vi "ClearFP.vi"(8 "error in (no error)":errorcluster, 9 "ConPaneMode?":bool=TRUE, 10 "ProjectItemRef":refnum<vi>, 11 "CS++Actor in":refnum<class "CS++Actor.lvclass">) -> (0 "error out":errorcluster, 3 "CS++Actor out":refnum<class "CS++Actor.lvclass">)   [LabVIEW 2016, in "CS++Actor.lvlib" / "CS++Actor.lvclass"]
doc: "This VI resets FP elements. All controls will be on the left side, all indicators on the right side."
uses:
  CS++Actor.lvclass
  <vilib>/Utility/traverseref.llb/TRef TravTarget.ctl
  <vilib>/Utility/miscctls.llb/LVRectTypeDef.ctl
  <vilib>/Utility/VariantDataType/Type.ctl
  <vilib>/Utility/VariantDataType/VariantType.lvlib
  <vilib>/Utility/Data Type/NI_Data Type.lvlib
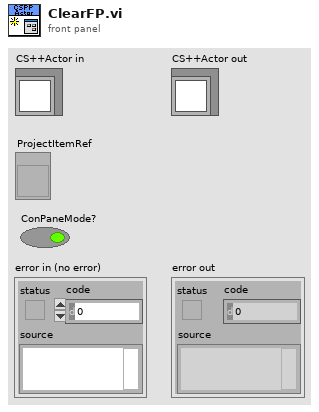
[diagram p1: front panel]
types:
  T1 = enum16{"Invalid Wire Rule", "Required", "Recommended", "Optional", "Dynamic Dispatch"}
  T2 = enum32{"Top Edges", "Vertical Centers", "Bottom Edges", "Left Edges", "Horizontal Centers", "Right Edges"}
  T3 = enum32{"Top Edges", "Vertical Centers", "Bottom Edges", "Vertical Gap", "Vertical Compress", "Left Edges", "Horizontal Centers", "Right Edges", "Horizontal Gap", "Horizontal Compress"}
  T4 = typedef "TRef TravTarget.ctl" = enum16{"FP", "BD", "Other"}
  T5 = typedef "LVRectTypeDef.ctl" = cluster{"Left":i16, "Top":i16, "Right":i16, "Bottom":i16}
  T6 = typedef "VariantType.lvlib/Type.ctl" = enum8{"Invalid Type", "Void", "I8", "I16", "I32", "I64", "U8", "U16", "U32", "U64", "Single Float", "Double Float", "Extended Float", "Single Complex", "Double Complex", "Extended Complex", "Enum U8", "Enum U16", "Enum U32", "Enum U64", "Single Float With Unit", "Double Float With Unit", "Extended Float With Unit", "Single Complex with Unit", "Double Complex with Unit", "Extended Complex with Unit", "Boolean", "String", "Path", "Picture", "Tag", "Array", "Cluster", "Variant", "LV Variant", "Waveform", "Timestamp", "Digital Waveform", "Digital Data", "ExpressData", "Refnum", "External Data", "VI", "Poly VI", "LabVIEW Class Instance", "Fixed Point"}
  T7 = enum16{"Invalid Wire Rule", "Required", "Recommended", "Optional", "Dynamic Dispatch"}[]
  T8 = typedef "NI_Data Type.lvlib/Data Type.ctl" = enum8{"Invalid Type", "Void", "I8", "I16", "I32", "I64", "U8", "U16", "U32", "U64", "Single Float", "Double Float", "Extended Float", "Single Complex", "Double Complex", "Extended Complex", "Enum U8", "Enum U16", "Enum U32", "Enum U64", "Single Float With Unit", "Double Float With Unit", "Extended Float With Unit", "Single Complex with Unit", "Double Complex with Unit", "Extended Complex with Unit", "Boolean", "String", "Path", "Picture", "Tag", "Array", "Cluster", "Variant", "LV Variant", "Waveform", "Timestamp", "Digital Waveform", "Digital Data", "ExpressData", "Refnum", "External Data", "VI", "Poly VI", "LabVIEW Class Instance", "Fixed Point"}
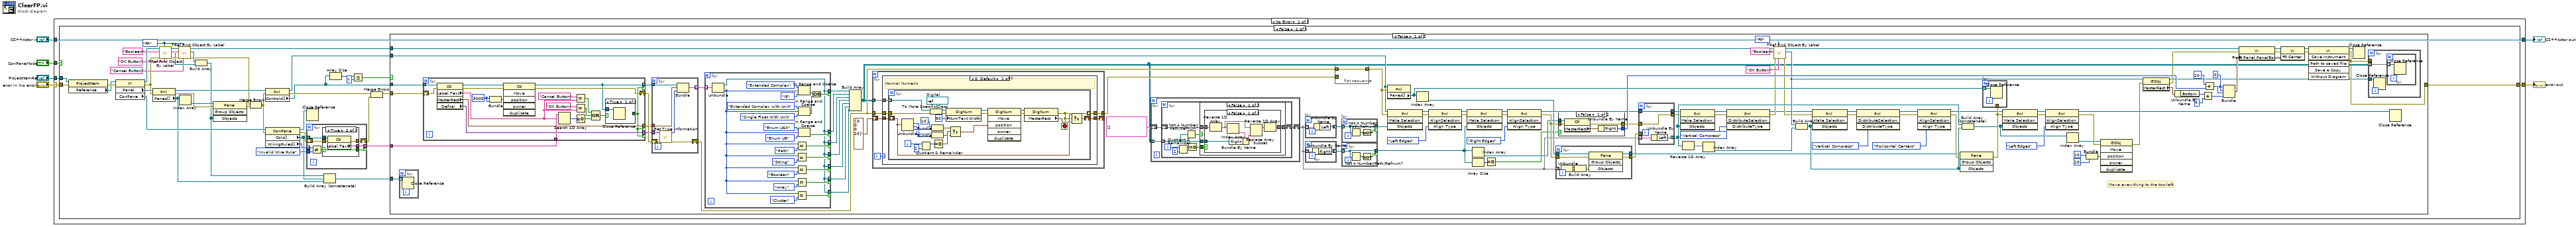
[diagram p0: block diagram]
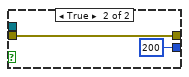
[diagram p2: hidden frame]
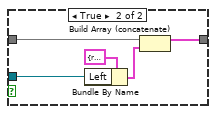
[diagram p3: hidden frame]
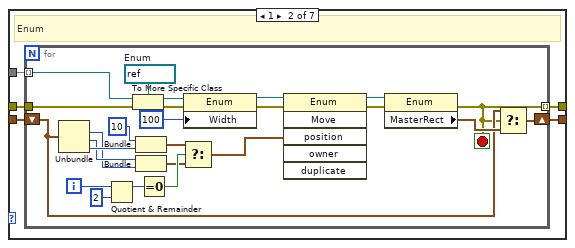
[diagram p5: hidden frame]
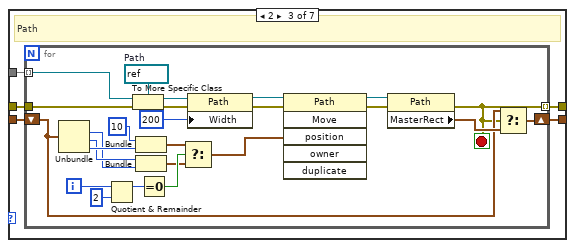
[diagram p6: hidden frame]
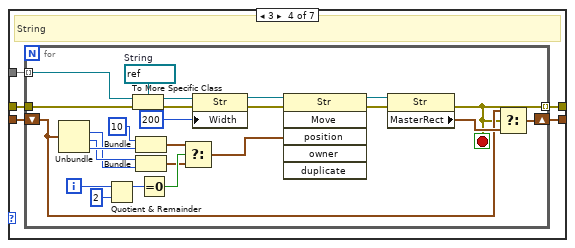
[diagram p7: hidden frame]
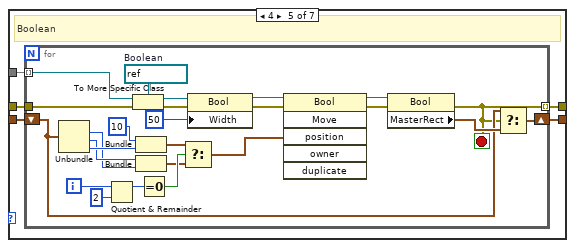
[diagram p8: hidden frame]
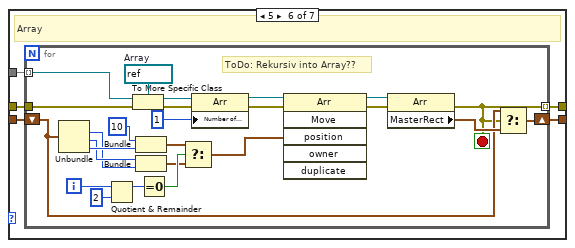
[diagram p9: hidden frame]
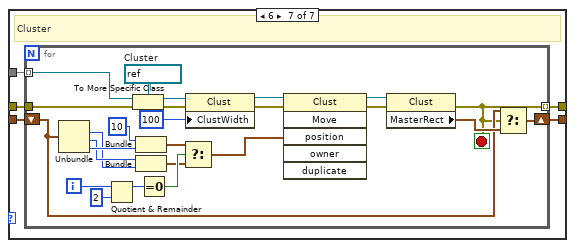
[diagram p10: hidden frame]
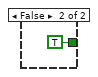
[diagram p11: hidden frame]
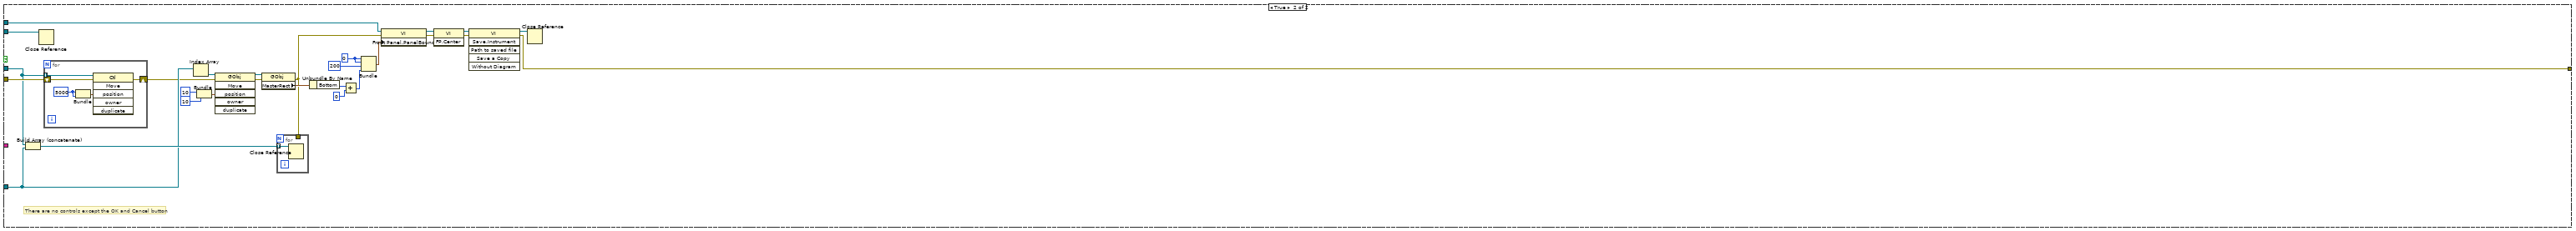
[diagram p12: hidden frame]
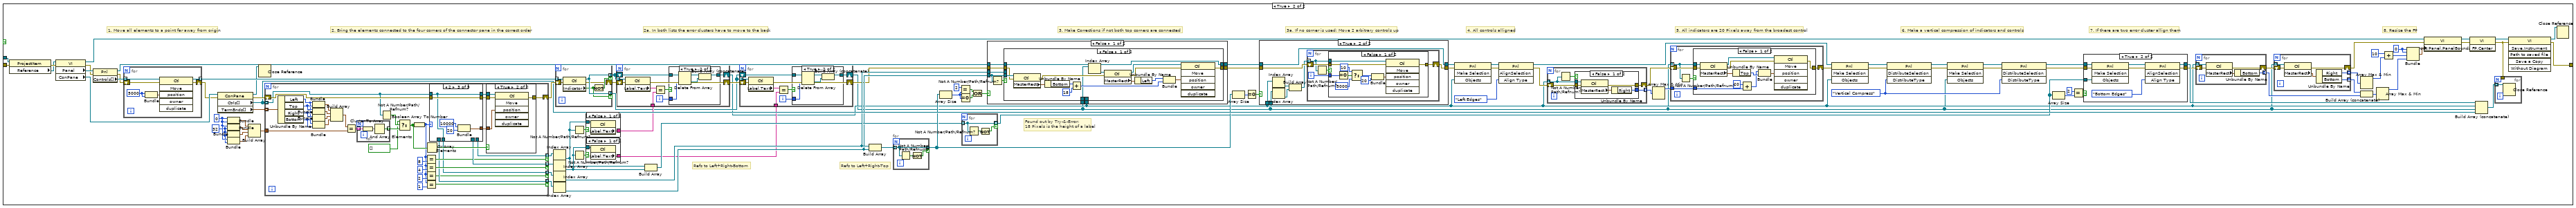
[diagram p14: hidden frame]
diagram:
  n1 = case shown="No Error" "error in (no error)" {
    selector: "error in (no error)" -> [w9 w872]
    tunnel: [w10 w872] -> w5
    tunnel: [w11 w871] -> w3
    tunnel: "CS++Actor in" -> [w11 w871]
    tunnel: "ProjectItemRef" -> [w8 _]
    tunnel: "ConPaneMode?" -> [w7 _]
    frame No Error {
      n2 = case shown="False" w7 {
        tunnel: [w42 w577] -> w10
        tunnel: w9 -> [w40 w576]
        tunnel: w8 -> [w41 w573]
        frame False {
          w31 = "Boolean" ("Class Name")
          w32 = TRef_TravTarget."FP" ("Traverse Target")
          n3 = property class="ProjectItem"(reference=w41, error in=w40) -> (error out=w39:errorcluster, "Reference"=w38:refnum<vi>)  [unwired: 1 out]
          n4 = property class="VI"(reference=w38, error in=w39) -> (reference out=w37:refnum<vi>, error out=w23:errorcluster, "Panel"=w29:refnum<vi>, "ConPane"=w43:refnum<vi>)
          n5 = property class="Pnl"(reference=w29, error in=w23) -> (reference out=w28:refnum<vi>, error out=w26:errorcluster, "Panes[]"=w19:refnum<vi>[])
          n6 = call <vilib>:"TRef Find Object By Label.vi"("Label"="OK Button", "Traverse Target"=w32, "error in (no error)"=w23, "Class Name"=w31, "VI Ref"=w37) -> ("error out"=w33:errorcluster, "Found Obj Ref"=w24:refnum<vi>, "dup VI Ref"=w35:refnum<vi>)  [unwired: 3 in, 1 out]
          n7 = call <vilib>:"TRef Find Object By Label.vi"("Label"="Cancel Button", "Traverse Target"=w32, "error in (no error)"=w33, "Class Name"=w31, "VI Ref"=w35) -> ("error out"=w21:errorcluster, "Found Obj Ref"=w25:refnum<vi>, "dup VI Ref"=w34:refnum<vi>)  [unwired: 3 in, 1 out]
          n8 = Index Array(array=w19) -> (element=w27:refnum<vi>)  [unwired: 1 in]
          n9 = Build Array(w25, w24) -> (w13:refnum<vi>[])
          n10 = invoke class="Pane" method="Group Objects"(reference=w27, error in=w26, "Objects"=w13) -> (error out=w22:errorcluster)  [unwired: 1 in, 3 out]
          n11 = Merge Errors(w21, w22) -> (w20:errorcluster)
          n12 = property class="Pnl"(reference=w28, error in=w20) -> (reference out=w51:refnum<vi>, error out=w45:errorcluster, "Controls[]"=w18:refnum<vi>[])
          n13 = property class="ConPane"(reference=w43, error in=w20) -> (reference out=w48:refnum<vi>, error out=w44:errorcluster, "Ctrls[]"=w12:refnum<vi>[], "WiringRules[]"=w49:T7)
          n14 = Close Reference(reference=w48) -> ()  [unwired: 1 in, 1 out]
          n15 = for {
            tunnel: w12 -> [w525] mode=indexing
            shift-right: [w523] -> w47
            shift-left: w44 -> [w524]
            tunnel: [w522] -> w52 mode=indexing if=w518
            tunnel: w49 -> [w520] mode=indexing
            tunnel: T1."Invalid Wire Rule" ("Wire Rule") -> [w519]
            n16 = Not Equal?(x=w520, y=w519) -> (x != y?=w521:bool)
            n17 = case shown="True" w521 {
              selector: w521 -> [w526 w528]
              tunnel: w525 -> [_ w532]
              tunnel: w524 -> [w527 w531]
              tunnel: [w527 w530] -> w523
              tunnel: [_ w529] -> w522
              tunnel: [w526 w528] -> w518
              frame False {
              }
              frame True {
                n18 = property class="Ctl"(reference=w532, error in=w531) -> (error out=w530:errorcluster, "Label.Text"=w529:string)  [unwired: 1 out]
              }
            }
          }
          n19 = Build Array (concatenate)(w13, w12, w19) -> (w14:refnum<vi>[])
          n20 = Array Size(array=w18) -> (size(s)=w17:i32)
          n21 = Less Or Equal?(x=w17, y=7) -> (x <= y?=w15:bool)
          n22 = Merge Errors(w45, w47) -> (w46:errorcluster)
          n23 = case shown="False" w15 {
            tunnel: w52 -> [w148 _]
            tunnel: w51 -> [w100 w492]
            tunnel: w46 -> [w71 w487]
            tunnel: [w70 w490] -> w42
            tunnel: w34 -> [w55 w496]
            tunnel: w18 -> [w54 w485]
            tunnel: w14 -> [w53 w488]
            frame False {
              w140 = i16 0 ("y")
              # "Move everything to the top-left"
              n24 = for {
                tunnel: w53 -> [w154] mode=indexing
                n25 = Close Reference(reference=w154) -> ()  [unwired: 1 in, 1 out]
              }
              n26 = for {
                tunnel: w54 -> [w482] mode=indexing
                shift-right: [w474] -> w75
                shift-left: w71 -> [w481]
                tunnel: w148 -> [w480]
                tunnel: [w475] -> w74 mode=indexing if=w471
                tunnel: [w473] -> w73 mode=indexing if=w471
                tunnel: [w472] -> w72 mode=indexing if=w471
                w479 = i16 5000 ("x")
                n27 = property class="Ctl"(reference=w482, error in=w481) -> (reference out=w476:refnum<vi>, error out=w477:errorcluster, "Label.Text"=w469:string, "MasterRect"=w473:T5, "DefVal"=w472:variant)
                n28 = Bundle("x"=w479, "x"=w479) -> (w478:cluster{"x":i16, "x":i16})  [unwired: 1 in]
                n29 = invoke class="Ctl" method="Move"(reference=w476, error in=w477, "position"=w478) -> (reference out=w475:refnum<vi>, error out=w474:errorcluster)  [unwired: 3 in, 4 out]
                n30 = Search 1D Array(1D array=w480, element=w469) -> (index of element=w470:i32)  [unwired: 1 in]
                n31 = Equal?(x="Cancel Button", y=w469) -> (x = y?=w468:bool)
                n32 = Equal?(x="OK Button", y=w469) -> (x = y?=w467:bool)
                n33 = Greater Or Equal To 0?(x=w470) -> (x >= 0?=w466:bool)
                n34 = Compound Arithmetic op=OR(w468, w467, w466) -> (w465:bool)
                n35 = case shown="True" w465 {
                  tunnel: w475 -> [w483 _]
                  tunnel: [_ TRUE] -> w471
                  frame True {
                    n36 = Close Reference(reference=w483) -> ()  [unwired: 1 in, 1 out]
                  }
                  frame False {
                  }
                }
              }
              n37 = for {
                tunnel: w72 -> [w462] mode=indexing
                tunnel: w73 -> [w460] mode=indexing
                tunnel: w74 -> [w461] mode=indexing
                tunnel: [w459] -> w76 mode=indexing
                shift-right: [w457] -> w98
                shift-left: w75 -> [w458]
                n38 = call <vilib>:"Get Type Information.vi"("error in (no error)"=w458, "Variant"=w462) -> ("error out"=w457:errorcluster, "Type"=w456:T8)  [unwired: 5 in, 3 out]
                n39 = Bundle(w461, "MasterRect"=w460, "Type"=w456) -> (w459:cluster{refnum<vi>, "MasterRect":T5, "Type":T8})  [unwired: 1 in]
              }
              n40 = for {
                tunnel: w76 -> [w435] mode=indexing
                tunnel: [w433] -> w77 mode=indexing if=w449
                tunnel: [w433] -> w78 mode=indexing if=w446
                tunnel: [w433] -> w79 mode=indexing if=w436
                tunnel: [w433] -> w82 mode=indexing if=w444
                tunnel: [w433] -> w83 mode=indexing if=w441
                tunnel: [w433] -> w84 mode=indexing if=w440
                tunnel: [w433] -> w81 mode=indexing if=w434
                n41 = Unbundle(w435) -> (w433:refnum<vi>, "Type"=w437:T8)  [unwired: 1 out]
                n42 = Equal?(x=w437, y=Type."Path" ("Type Enum")) -> (x = y?=w436:bool)
                n43 = Equal?(x=w437, y=Type."String" ("Type Enum")) -> (x = y?=w434:bool)
                n44 = Equal?(x=w437, y=Type."Boolean" ("Type Enum")) -> (x = y?=w444:bool)
                n45 = Equal?(x=w437, y=Type."Array" ("Type Enum")) -> (x = y?=w441:bool)
                n46 = Equal?(x=w437, y=Type."Cluster" ("Type Enum")) -> (x = y?=w440:bool)
                n47 = In Range and Coerce(upper limit=Type."Extended Complex" ("Type Enum"), x=w437, lower limit=Type."I8" ("Type Enum")) -> (In Range?=w451:bool)  [unwired: 1 out]
                n48 = In Range and Coerce(upper limit=Type."Extended Complex with Unit" ("Type Enum"), x=w437, lower limit=Type."Single Float With Unit" ("Type Enum")) -> (In Range?=w450:bool)  [unwired: 1 out]
                n49 = In Range and Coerce(upper limit=Type."Enum U64" ("Type Enum"), x=w437, lower limit=Type."Enum U8" ("Type Enum")) -> (In Range?=w446:bool)  [unwired: 1 out]
                n50 = Or(x=w451, y=w450) -> (x .or. y?=w449:bool)
              }
              n51 = Build Array(w77, w78, w79, w81, w82, w83, w84) -> (w85:refnum<vi>[][])
              n52 = for {
                tunnel: w85 -> [w221] mode=indexing
                shift-right: [w218] -> _
                shift-left: T5 {"Left"=0, "Top"=0, "Right"=0, "Bottom"=20} ("MasterRect") -> [w219]
                tunnel: w98 -> [w222]
                tunnel: [w217] -> w99 mode=concatenating
                i -> [w220]
                n53 = case shown="0, Default" w220 {
                  tunnel: w221 -> [w227 w257 w287 w317 w347 w377 w407]
                  tunnel: [w226 w256 w286 w316 w346 w376 w406] -> w217
                  tunnel: [w225 w255 w285 w315 w345 w375 w405] -> w218
                  tunnel: w222 -> [w224 w254 w284 w314 w344 w374 w404]
                  tunnel: w219 -> [w223 w253 w283 w313 w343 w373 w403]
                  frame 0, Default {
                    # "Normal Numeric"
                    n54 = for {
                      tunnel: w227 -> [w232] mode=indexing
                      shift-right: [w231] -> w225
                      shift-left: w223 -> [w229]
                      tunnel: w224 -> [w251]
                      tunnel: [w228] -> w226 mode=indexing
                      i -> [w252]
                      stop <- w228 stop-if-true
                      w233 = refnum<vi> refnum  # Digital
                      n55 = Unbundle(w229) -> ("Top"=w234:i16, "Right"=w235:i16, "Bottom"=w236:i16)  [unwired: 1 out]
                      n56 = Quotient & Remainder(x=w252, y=2) -> (x-y*floor(x/y)=w242:i32)  [unwired: 1 out]
                      n57 = To More Specific Class(target class=w233, reference=w232, error in=w251) -> (specific class reference=w249:refnum<vi>, error out=w248:errorcluster)
                      n58 = Bundle("Top"=i16 10, "Bottom"=w236) -> (w239:cluster{"Top":i16, "Bottom":i16})  [unwired: 1 in]
                      n59 = Bundle("Right"=w235, "Top"=w234) -> (w238:cluster{"Right":i16, "Top":i16})  [unwired: 1 in]
                      n60 = Equal To 0?(x=w242) -> (x = 0?=w241:bool)
                      n61 = property class="DigNum"(reference=w249, error in=w248, "NumText.Width"=u32 50 ("Numeric Text.Size:Width")) -> (reference out=w247:refnum<vi>, error out=w246:errorcluster)
                      n62 = Select(t=w239, s=w241, f=w238) -> (s? t:f=w240:cluster{"Right":i16, "Top":i16})
                      n63 = invoke class="DigNum" method="Move"(reference=w247, error in=w246, "position"=w240) -> (reference out=w244:refnum<vi>, error out=w243:errorcluster)  [unwired: 3 in, 4 out]
                      n64 = property class="DigNum"(reference=w244, error in=w243) -> (error out=w228:errorcluster, "MasterRect"=w230:T5)  [unwired: 1 out]
                      n65 = Select(t=w229, s=w228, f=w230) -> (s? t:f=w231:T5)
                    }
                  }
                  frame 1 {
                    # "Enum"
                    n66 = for {
                      tunnel: w257 -> [w262] mode=indexing
                      shift-right: [w261] -> w255
                      shift-left: w253 -> [w259]
                      tunnel: w254 -> [w281]
                      tunnel: [w258] -> w256 mode=indexing
                      i -> [w282]
                      stop <- w258 stop-if-true
                      w263 = refnum<vi> refnum  # Enum
                      n67 = Unbundle(w259) -> ("Top"=w264:i16, "Right"=w265:i16, "Bottom"=w266:i16)  [unwired: 1 out]
                      n68 = Quotient & Remainder(x=w282, y=2) -> (x-y*floor(x/y)=w272:i32)  [unwired: 1 out]
                      n69 = To More Specific Class(target class=w263, reference=w262, error in=w281) -> (specific class reference=w279:refnum<vi>, error out=w278:errorcluster)
                      n70 = Bundle("Top"=i16 10, "Bottom"=w266) -> (w269:cluster{"Top":i16, "Bottom":i16})  [unwired: 1 in]
                      n71 = Bundle("Right"=w265, "Top"=w264) -> (w268:cluster{"Right":i16, "Top":i16})  [unwired: 1 in]
                      n72 = Equal To 0?(x=w272) -> (x = 0?=w271:bool)
                      n73 = Select(t=w269, s=w271, f=w268) -> (s? t:f=w270:cluster{"Right":i16, "Top":i16})
                      n74 = property class="Enum"(reference=w279, error in=w278, "Width"=u32 100 ("Numeric Text.Size:Width")) -> (reference out=w277:refnum<vi>, error out=w276:errorcluster)
                      n75 = invoke class="Enum" method="Move"(reference=w277, error in=w276, "position"=w270) -> (reference out=w274:refnum<vi>, error out=w273:errorcluster)  [unwired: 3 in, 4 out]
                      n76 = property class="Enum"(reference=w274, error in=w273) -> (error out=w258:errorcluster, "MasterRect"=w260:T5)  [unwired: 1 out]
                      n77 = Select(t=w259, s=w258, f=w260) -> (s? t:f=w261:T5)
                    }
                  }
                  frame 2 {
                    # "Path"
                    n78 = for {
                      tunnel: w287 -> [w292] mode=indexing
                      shift-right: [w291] -> w285
                      shift-left: w283 -> [w289]
                      tunnel: w284 -> [w311]
                      tunnel: [w288] -> w286 mode=indexing
                      i -> [w312]
                      stop <- w288 stop-if-true
                      w293 = refnum<vi> refnum  # Path
                      n79 = Unbundle(w289) -> ("Top"=w294:i16, "Right"=w295:i16, "Bottom"=w296:i16)  [unwired: 1 out]
                      n80 = Quotient & Remainder(x=w312, y=2) -> (x-y*floor(x/y)=w302:i32)  [unwired: 1 out]
                      n81 = To More Specific Class(target class=w293, reference=w292, error in=w311) -> (specific class reference=w309:refnum<vi>, error out=w308:errorcluster)
                      n82 = Bundle("Top"=i16 10, "Bottom"=w296) -> (w299:cluster{"Top":i16, "Bottom":i16})  [unwired: 1 in]
                      n83 = Bundle("Right"=w295, "Top"=w294) -> (w298:cluster{"Right":i16, "Top":i16})  [unwired: 1 in]
                      n84 = Equal To 0?(x=w302) -> (x = 0?=w301:bool)
                      n85 = Select(t=w299, s=w301, f=w298) -> (s? t:f=w300:cluster{"Right":i16, "Top":i16})
                      n86 = property class="Path"(reference=w309, error in=w308, "Width"=u32 200 ("Numeric Text.Size:Width")) -> (reference out=w307:refnum<vi>, error out=w306:errorcluster)
                      n87 = invoke class="Path" method="Move"(reference=w307, error in=w306, "position"=w300) -> (reference out=w304:refnum<vi>, error out=w303:errorcluster)  [unwired: 3 in, 4 out]
                      n88 = property class="Path"(reference=w304, error in=w303) -> (error out=w288:errorcluster, "MasterRect"=w290:T5)  [unwired: 1 out]
                      n89 = Select(t=w289, s=w288, f=w290) -> (s? t:f=w291:T5)
                    }
                  }
                  frame 3 {
                    # "String"
                    n90 = for {
                      tunnel: w317 -> [w322] mode=indexing
                      shift-right: [w321] -> w315
                      shift-left: w313 -> [w319]
                      tunnel: w314 -> [w341]
                      tunnel: [w318] -> w316 mode=indexing
                      i -> [w342]
                      stop <- w318 stop-if-true
                      w323 = refnum<vi> refnum  # String
                      n91 = Unbundle(w319) -> ("Top"=w324:i16, "Right"=w325:i16, "Bottom"=w326:i16)  [unwired: 1 out]
                      n92 = Quotient & Remainder(x=w342, y=2) -> (x-y*floor(x/y)=w332:i32)  [unwired: 1 out]
                      n93 = To More Specific Class(target class=w323, reference=w322, error in=w341) -> (specific class reference=w339:refnum<vi>, error out=w338:errorcluster)
                      n94 = Bundle("Top"=i16 10, "Bottom"=w326) -> (w329:cluster{"Top":i16, "Bottom":i16})  [unwired: 1 in]
                      n95 = Bundle("Right"=w325, "Top"=w324) -> (w328:cluster{"Right":i16, "Top":i16})  [unwired: 1 in]
                      n96 = Equal To 0?(x=w332) -> (x = 0?=w331:bool)
                      n97 = Select(t=w329, s=w331, f=w328) -> (s? t:f=w330:cluster{"Right":i16, "Top":i16})
                      n98 = property class="Str"(reference=w339, error in=w338, "Width"=u32 200 ("Numeric Text.Size:Width")) -> (reference out=w337:refnum<vi>, error out=w336:errorcluster)
                      n99 = invoke class="Str" method="Move"(reference=w337, error in=w336, "position"=w330) -> (reference out=w334:refnum<vi>, error out=w333:errorcluster)  [unwired: 3 in, 4 out]
                      n100 = property class="Str"(reference=w334, error in=w333) -> (error out=w318:errorcluster, "MasterRect"=w320:T5)  [unwired: 1 out]
                      n101 = Select(t=w319, s=w318, f=w320) -> (s? t:f=w321:T5)
                    }
                  }
                  frame 4 {
                    # "Boolean"
                    n102 = for {
                      tunnel: w347 -> [w352] mode=indexing
                      shift-right: [w351] -> w345
                      shift-left: w343 -> [w349]
                      tunnel: w344 -> [w371]
                      tunnel: [w348] -> w346 mode=indexing
                      i -> [w372]
                      stop <- w348 stop-if-true
                      w353 = refnum<vi> refnum  # Boolean
                      n103 = Unbundle(w349) -> ("Top"=w354:i16, "Right"=w355:i16, "Bottom"=w356:i16)  [unwired: 1 out]
                      n104 = Quotient & Remainder(x=w372, y=2) -> (x-y*floor(x/y)=w362:i32)  [unwired: 1 out]
                      n105 = To More Specific Class(target class=w353, reference=w352, error in=w371) -> (specific class reference=w369:refnum<vi>, error out=w368:errorcluster)
                      n106 = Bundle("Top"=i16 10, "Bottom"=w356) -> (w359:cluster{"Top":i16, "Bottom":i16})  [unwired: 1 in]
                      n107 = Bundle("Right"=w355, "Top"=w354) -> (w358:cluster{"Right":i16, "Top":i16})  [unwired: 1 in]
                      n108 = Equal To 0?(x=w362) -> (x = 0?=w361:bool)
                      n109 = Select(t=w359, s=w361, f=w358) -> (s? t:f=w360:cluster{"Right":i16, "Top":i16})
                      n110 = property class="Bool"(reference=w369, error in=w368, "Width"=u32 50 ("Numeric Text.Size:Width")) -> (reference out=w367:refnum<vi>, error out=w366:errorcluster)
                      n111 = invoke class="Bool" method="Move"(reference=w367, error in=w366, "position"=w360) -> (reference out=w364:refnum<vi>, error out=w363:errorcluster)  [unwired: 3 in, 4 out]
                      n112 = property class="Bool"(reference=w364, error in=w363) -> (error out=w348:errorcluster, "MasterRect"=w350:T5)  [unwired: 1 out]
                      n113 = Select(t=w349, s=w348, f=w350) -> (s? t:f=w351:T5)
                    }
                  }
                  frame 5 {
                    # "Array"
                    n114 = for {
                      tunnel: w377 -> [w382] mode=indexing
                      shift-right: [w381] -> w375
                      shift-left: w373 -> [w379]
                      tunnel: w374 -> [w401]
                      tunnel: [w378] -> w376 mode=indexing
                      i -> [w402]
                      stop <- w378 stop-if-true
                      w383 = refnum<vi> refnum  # Array
                      # "ToDo: Rekursiv into Array??"
                      n115 = Unbundle(w379) -> ("Top"=w384:i16, "Right"=w385:i16, "Bottom"=w386:i16)  [unwired: 1 out]
                      n116 = Quotient & Remainder(x=w402, y=2) -> (x-y*floor(x/y)=w392:i32)  [unwired: 1 out]
                      n117 = To More Specific Class(target class=w383, reference=w382, error in=w401) -> (specific class reference=w399:refnum<vi>, error out=w398:errorcluster)
                      n118 = Bundle("Top"=i16 10, "Bottom"=w386) -> (w389:cluster{"Top":i16, "Bottom":i16})  [unwired: 1 in]
                      n119 = Bundle("Right"=w385, "Top"=w384) -> (w388:cluster{"Right":i16, "Top":i16})  [unwired: 1 in]
                      n120 = Equal To 0?(x=w392) -> (x = 0?=w391:bool)
                      n121 = Select(t=w389, s=w391, f=w388) -> (s? t:f=w390:cluster{"Right":i16, "Top":i16})
                      n122 = property class="Arr"(reference=w399, error in=w398, "Number of Columns"=u32 1 ("Numeric Text.Size:Width")) -> (reference out=w397:refnum<vi>, error out=w396:errorcluster)
                      n123 = invoke class="Arr" method="Move"(reference=w397, error in=w396, "position"=w390) -> (reference out=w394:refnum<vi>, error out=w393:errorcluster)  [unwired: 3 in, 4 out]
                      n124 = property class="Arr"(reference=w394, error in=w393) -> (error out=w378:errorcluster, "MasterRect"=w380:T5)  [unwired: 1 out]
                      n125 = Select(t=w379, s=w378, f=w380) -> (s? t:f=w381:T5)
                    }
                  }
                  frame 6 {
                    # "Cluster"
                    n126 = for {
                      tunnel: w407 -> [w412] mode=indexing
                      shift-right: [w411] -> w405
                      shift-left: w403 -> [w409]
                      tunnel: w404 -> [w431]
                      tunnel: [w408] -> w406 mode=indexing
                      i -> [w432]
                      stop <- w408 stop-if-true
                      w413 = refnum<vi> refnum  # Cluster
                      n127 = Unbundle(w409) -> ("Top"=w414:i16, "Right"=w415:i16, "Bottom"=w416:i16)  [unwired: 1 out]
                      n128 = Quotient & Remainder(x=w432, y=2) -> (x-y*floor(x/y)=w422:i32)  [unwired: 1 out]
                      n129 = To More Specific Class(target class=w413, reference=w412, error in=w431) -> (specific class reference=w429:refnum<vi>, error out=w428:errorcluster)
                      n130 = Bundle("Top"=i16 10, "Bottom"=w416) -> (w419:cluster{"Top":i16, "Bottom":i16})  [unwired: 1 in]
                      n131 = Bundle("Right"=w415, "Top"=w414) -> (w418:cluster{"Right":i16, "Top":i16})  [unwired: 1 in]
                      n132 = Equal To 0?(x=w422) -> (x = 0?=w421:bool)
                      n133 = Select(t=w419, s=w421, f=w418) -> (s? t:f=w420:cluster{"Right":i16, "Top":i16})
                      n134 = property class="Clust"(reference=w429, error in=w428, "ClustWidth"=u32 100 ("Numeric Text.Size:Width")) -> (reference out=w427:refnum<vi>, error out=w426:errorcluster)
                      n135 = invoke class="Clust" method="Move"(reference=w427, error in=w426, "position"=w420) -> (reference out=w424:refnum<vi>, error out=w423:errorcluster)  [unwired: 3 in, 4 out]
                      n136 = property class="Clust"(reference=w424, error in=w423) -> (error out=w408:errorcluster, "MasterRect"=w410:T5)  [unwired: 1 out]
                      n137 = Select(t=w409, s=w408, f=w410) -> (s? t:f=w411:T5)
                    }
                  }
                }
              }
              n138 = for {
                tunnel: w85 -> [w188] mode=indexing
                shift-right: [w186] -> w103
                shift-left: cluster{"Left":refnum<vi>, "Right":refnum<vi>}[] [] -> [w187]
                n139 = for {
                  tunnel: w188 -> [w190] mode=indexing
                  shift-right: [w191] -> w186
                  shift-left: w187 -> [w192]
                  i -> [w194]
                  n140 = Quotient & Remainder(x=w194, y=2) -> (x-y*floor(x/y)=w195:i32)  [unwired: 1 out]
                  n141 = Not A Number/Path/Refnum?(number/path/refnum=w190) -> (NaN/Path/Refnum?=w189:bool)
                  n142 = Equal To 0?(x=w195) -> (x = 0?=w193:bool)
                  n143 = case shown="False" w189 {
                    tunnel: w193 -> [w200 _]
                    tunnel: w192 -> [w199 w213]
                    tunnel: [w198 w213] -> w191
                    tunnel: w190 -> [w197 _]
                    frame False {
                      n144 = case shown="False" w200 {
                        tunnel: w199 -> [w207 w212]
                        tunnel: [w204 w211] -> w198
                        tunnel: w197 -> [w201 w210]
                        frame False {
                          n145 = Reverse 1D Array(array=w207) -> (reversed array=w206:cluster{"Left":refnum<vi>, "Right":refnum<vi>}[])
                          n146 = Index Array(array=w206) -> (element=w203:cluster{"Left":refnum<vi>, "Right":refnum<vi>})  [unwired: 1 in]
                          n147 = Bundle By Name(cluster=w203, "Right"=w201) -> (w202:cluster{"Left":refnum<vi>, "Right":refnum<vi>})
                          n148 = Replace Array Subset(array=w206, new element=w202) -> (w205:cluster{"Left":refnum<vi>, "Right":refnum<vi>}[])  [unwired: 1 in]
                          n149 = Reverse 1D Array(array=w205) -> (reversed array=w204:cluster{"Left":refnum<vi>, "Right":refnum<vi>}[])
                        }
                        frame True {
                          n150 = Bundle By Name(cluster=cluster{"Left":refnum<vi>, "Right":refnum<vi>} {"Left"=refnum, "Right"=refnum}, "Left"=w210) -> (w208:cluster{"Left":refnum<vi>, "Right":refnum<vi>})
                          n151 = Build Array (concatenate)(w212, w208) -> (w211:cluster{"Left":refnum<vi>, "Right":refnum<vi>}[])
                        }
                      }
                    }
                    frame True {
                    }
                  }
                }
              }
              n152 = for {
                tunnel: w103 -> [w185] mode=indexing
                tunnel: [w184] -> w96 mode=indexing
                n153 = Unbundle By Name(w185) -> ("Left"=w184:refnum<vi>)
              }
              n154 = for {
                tunnel: w103 -> [w183] mode=indexing
                tunnel: [w182] -> w95 mode=indexing
                n155 = Unbundle By Name(w183) -> ("Right"=w182:refnum<vi>)
              }
              n156 = flat-sequence {
                tunnel: w98 -> [w175]
                tunnel: [w175] -> w101
                tunnel: w99 -> [_]
                frame #0 {
                }
              }
              n157 = for {
                tunnel: w96 -> [w176] mode=indexing
                tunnel: [w176] -> w97 mode=indexing if=w177
                n158 = Not A Number/Path/Refnum?(number/path/refnum=w176) -> (NaN/Path/Refnum?=w178:bool)
                n159 = Not(x=w178) -> (.not. x?=w177:bool)
              }
              n160 = for {
                tunnel: w95 -> [w179] mode=indexing
                tunnel: [w179] -> w67 mode=indexing if=w180
                n161 = Not A Number/Path/Refnum?(number/path/refnum=w179) -> (NaN/Path/Refnum?=w181:bool)
                n162 = Not(x=w181) -> (.not. x?=w180:bool)
              }
              n163 = property class="Pnl"(reference=w100, error in=w101) -> ("Panes[]"=w150:refnum<vi>[])  [unwired: 2 out]
              n164 = invoke class="Pnl" method="Make Selection"(reference=w100, error in=w101, "Objects"=w97) -> (reference out=w87:refnum<vi>, error out=w88:errorcluster)  [unwired: 1 in, 2 out]
              n165 = Index Array(array=w150) -> (element=w102:refnum<vi>)  [unwired: 1 in]
              n166 = invoke class="Pnl" method="AlignSelection"(reference=w87, error in=w88, "Align Type"=T2."Left Edges") -> (reference out=w93:refnum<vi>, error out=w94:errorcluster)  [unwired: 1 in, 2 out]
              n167 = invoke class="Pnl" method="Make Selection"(reference=w93, error in=w94, "Objects"=w67) -> (reference out=w90:refnum<vi>, error out=w91:errorcluster)  [unwired: 1 in, 2 out]
              n168 = Index Array(array=w67) -> (element=w68:refnum<vi>)  [unwired: 1 in]
              n169 = Array Size(array=w67) -> (size(s)=w66:i32)
              n170 = Equal To 0?(x=w66) -> (x = 0?=w65:bool)
              n171 = invoke class="Pnl" method="AlignSelection"(reference=w90, error in=w91, "Align Type"=T2."Right Edges") -> (reference out=w104:refnum<vi>, error out=w141:errorcluster)  [unwired: 1 in, 2 out]
              n172 = for {
                tunnel: w103 -> [w173] mode=indexing
                tunnel: w102 -> [w174]
                tunnel: w141 -> [w169]
                tunnel: [w168] -> w110
                tunnel: [w167] -> w125
                n173 = Unbundle(w173) -> ("Left"=w172:refnum<vi>, "Right"=w171:refnum<vi>)
                n174 = Build Array(w172, w171) -> (w170:refnum<vi>[])
                n175 = invoke class="Pane" method="Group Objects"(reference=w174, error in=w169, "Objects"=w170) -> (reference out=w167:refnum<vi>, error out=w168:errorcluster)  [unwired: 1 in, 2 out]
              }
              n176 = case shown="False" w65 {
                tunnel: [w159 i16 200 ("Right")] -> w145
                tunnel: [w157 w161] -> w142
                tunnel: w141 -> [w156 w161]
                tunnel: w68 -> [w155 _]
                frame False {
                  n177 = property class="Ctl"(reference=w155, error in=w156) -> (error out=w157:errorcluster, "MasterRect"=w158:T5)  [unwired: 1 out]
                  n178 = Unbundle By Name(w158) -> ("Right"=w159:i16)
                }
                frame True {
                }
              }
              n179 = for {
                tunnel: w103 -> [w166] mode=indexing
                tunnel: w104 -> [w165]
                tunnel: [w165] -> w105
                tunnel: w142 -> [w163]
                tunnel: [w164] -> w131 mode=indexing
                tunnel: [w163] -> w106
                tunnel: w110 -> [_]
                n180 = Unbundle By Name(w166) -> ("Left"=w164:refnum<vi>)
              }
              n181 = invoke class="Pnl" method="Make Selection"(reference=w105, error in=w106, "Objects"=w131) -> (reference out=w107:refnum<vi>, error out=w108:errorcluster)  [unwired: 1 in, 2 out]
              n182 = Reverse 1D Array(array=w131) -> (reversed array=w119:refnum<vi>[])
              n183 = Index Array(array=w119) -> (element=w120:refnum<vi>)  [unwired: 1 in]
              n184 = invoke class="Pnl" method="DistributeSelection"(reference=w107, error in=w108, "DistributeType"=T3."Vertical Compress") -> (reference out=w111:refnum<vi>, error out=w112:errorcluster)  [unwired: 1 in, 2 out]
              n185 = call <vilib>:"TRef Find Object By Label.vi"("Label"="OK Button", "Traverse Target"=TRef_TravTarget."FP", "error in (no error)"=w112, "Class Name"="Boolean", "VI Ref"=w55) -> ("error out"=w124:errorcluster, "Found Obj Ref"=w133:refnum<vi>, "dup VI Ref"=w132:refnum<vi>)  [unwired: 3 in, 1 out]
              n186 = Build Array(w133, w120) -> (w130:refnum<vi>[])
              n187 = invoke class="Pnl" method="Make Selection"(reference=w111, error in=w124, "Objects"=w130) -> (reference out=w116:refnum<vi>, error out=w117:errorcluster)  [unwired: 1 in, 2 out]
              n188 = invoke class="Pnl" method="DistributeSelection"(reference=w116, error in=w117, "DistributeType"=T3."Vertical Compress") -> (reference out=w121:refnum<vi>, error out=w122:errorcluster)  [unwired: 1 in, 2 out]
              n189 = invoke class="Pnl" method="AlignSelection"(reference=w121, error in=w122, "Align Type"=T2."Horizontal Centers") -> (reference out=w129:refnum<vi>, error out=w126:errorcluster)  [unwired: 1 in, 2 out]
              n190 = invoke class="Pane" method="Group Objects"(reference=w125, error in=w126, "Objects"=w130) -> (error out=w149:errorcluster)  [unwired: 1 in, 3 out]
              n191 = Build Array (concatenate)(w131, w130) -> (w59:refnum<vi>[])
              n192 = for {
                tunnel: w149 -> [_]
                tunnel: w150 -> [w162] mode=indexing
                n193 = Close Reference(reference=w162) -> ()  [unwired: 1 in, 1 out]
              }
              n194 = invoke class="Pnl" method="Make Selection"(reference=w129, error in=w149, "Objects"=w59) -> (reference out=w127:refnum<vi>, error out=w128:errorcluster)  [unwired: 1 in, 2 out]
              n195 = invoke class="Pnl" method="AlignSelection"(reference=w127, error in=w128, "Align Type"=T2."Left Edges") -> (reference out=w63:refnum<vi>, error out=w58:errorcluster)  [unwired: 1 in, 2 out]
              n196 = Index Array(array=w59) -> (element=w57:refnum<vi>)  [unwired: 1 in]
              n197 = Bundle("Top"=i16 10, "Top"=i16 10) -> (w61:cluster{"Top":i16, "Top":i16})  [unwired: 1 in]
              n198 = invoke class="GObj" method="Move"(reference=w57, error in=w58, "position"=w61) -> (error out=w62:errorcluster)  [unwired: 3 in, 5 out]
              n199 = property class="GObj"(reference=w133, error in=w62) -> (reference out=w134:refnum<vi>, error out=w69:errorcluster, "MasterRect"=w135:T5)
              n200 = Unbundle By Name(w135) -> ("Bottom"=w136:i16)
              n201 = Add(x=w136, y=i16 4) -> (x+y=w139:i16)
              n202 = Add(x=i16 10 ("y"), y=w145) -> (x+y=w143:i16)
              n203 = Bundle("y"=w140, "y"=w140, w143, w139) -> (w138:cluster{"y":i16, "y":i16, i16, i16})  [unwired: 1 in]
              n204 = property class="VI"(reference=w132, error in=w69, "Front Panel.PanelBounds"=w138) -> (reference out=w146:refnum<vi>, error out=w147:errorcluster)
              n205 = invoke class="VI" method="FP.Center"(reference=w146, error in=w147) -> (reference out=w151:refnum<vi>, error out=w153:errorcluster)  [unwired: 1 in, 1 out]
              n206 = invoke class="VI" method="Save.Instrument"(reference=w151, error in=w153) -> (reference out=w152:refnum<vi>, error out=w70:errorcluster)  [unwired: 4 in, 4 out]
              n207 = Close Reference(reference=w152) -> ()  [unwired: 1 in, 1 out]
              n208 = for {
                tunnel: w85 -> [w215] mode=indexing
                tunnel: w70 -> [_]
                tunnel: w134 -> [w214]
                n209 = Close Reference(reference=w214) -> ()  [unwired: 1 in, 1 out]
                n210 = for {
                  tunnel: w215 -> [w216] mode=indexing
                  n211 = Close Reference(reference=w216) -> ()  [unwired: 1 in, 1 out]
                }
              }
              n212 = Close Reference(reference=w63) -> ()  [unwired: 1 in, 1 out]
            }
            frame True {
              w497 = i16 0 ("y")
              # "There are no controls except the OK and Cancel button"
              n213 = Build Array (concatenate)(w485, w488) -> (w489:refnum<vi>[])
              n214 = Close Reference(reference=w492) -> ()  [unwired: 1 in, 1 out]
              n215 = for {
                shift-right: [w514] -> w486
                shift-left: w487 -> [w513]
                tunnel: w485 -> [w512] mode=indexing
                w515 = i16 5000 ("x")
                n216 = Bundle("x"=w515, "x"=w515) -> (w516:cluster{"x":i16, "x":i16})  [unwired: 1 in]
                n217 = invoke class="Ctl" method="Move"(reference=w512, error in=w513, "position"=w516) -> (error out=w514:errorcluster)  [unwired: 3 in, 5 out]
              }
              n218 = Index Array(array=w488) -> (element=w495:refnum<vi>)  [unwired: 1 in]
              n219 = Bundle("Top"=i16 10, "Top"=i16 10) -> (w510:cluster{"Top":i16, "Top":i16})  [unwired: 1 in]
              n220 = invoke class="GObj" method="Move"(reference=w495, error in=w486, "position"=w510) -> (reference out=w494:refnum<vi>, error out=w511:errorcluster)  [unwired: 3 in, 4 out]
              n221 = property class="GObj"(reference=w494, error in=w511) -> (error out=w491:errorcluster, "MasterRect"=w507:T5)  [unwired: 1 out]
              n222 = for {
                tunnel: w489 -> [w517] mode=indexing
                tunnel: w491 -> [_]
                n223 = Close Reference(reference=w517) -> ()  [unwired: 1 in, 1 out]
              }
              n224 = Unbundle By Name(w507) -> ("Bottom"=w504:i16)
              n225 = Add(x=w504, y=i16 0) -> (x+y=w506:i16)
              n226 = Bundle("y"=w497, "y"=w497, "y"=i16 200, w506) -> (w498:cluster{"y":i16, "y":i16, "y":i16, i16})  [unwired: 1 in]
              n227 = property class="VI"(reference=w496, error in=w491, "Front Panel.PanelBounds"=w498) -> (reference out=w499:refnum<vi>, error out=w500:errorcluster)
              n228 = invoke class="VI" method="FP.Center"(reference=w499, error in=w500) -> (reference out=w501:refnum<vi>, error out=w502:errorcluster)  [unwired: 1 in, 1 out]
              n229 = invoke class="VI" method="Save.Instrument"(reference=w501, error in=w502) -> (reference out=w503:refnum<vi>, error out=w490:errorcluster)  [unwired: 4 in, 4 out]
              n230 = Close Reference(reference=w503) -> ()  [unwired: 1 in, 1 out]
            }
          }
        }
        frame True {
          w594 = i16 0 ("x")
          w611 = i16 32
          w612 = i16 0
          w619 = T3."Vertical Compress" ("DistributeType")
          # "Found out by Try-&-Error: \n18 Pixels is the height of a label"
          # "2a. In both lists the error clusters have to move to the back"
          # "3a. If no corner is used: Move 2 arbitrary controls up"
          # "3. Make Corrections if not both top corners are connected"
          # "Refs to Left+Right-Top"
          # "Refs to Left+Right-Bottom"
          # "8. Resize the FP"
          # "7. If there are two error cluster allign them"
          # "2. Bring the elements connected to the four corners of the connector pane in the correct order"
          # "1. Move all elements to a point far away from origin"
          # "6. Make a vertical compression of indicators and controls"
          # "5. All indicators are 20 Pixels away from the broadest control"
          # "4. All controls alligned"
          n231 = property class="ProjectItem"(reference=w573, error in=w576) -> (error out=w575:errorcluster, "Reference"=w574:refnum<vi>)  [unwired: 1 out]
          n232 = property class="VI"(reference=w574, error in=w575) -> (reference out=w595:refnum<vi>, error out=w632:errorcluster, "Panel"=w633:refnum<vi>, "ConPane"=w615:refnum<vi>)
          n233 = property class="Pnl"(reference=w633, error in=w632) -> (reference out=w565:refnum<vi>, error out=w617:errorcluster, "Controls[]"=w618:refnum<vi>[])
          n234 = for {
            tunnel: w618 -> [w835] mode=indexing
            shift-right: [w833] -> w605
            shift-left: w617 -> [w834]
            tunnel: [w832] -> w616 mode=indexing
            w830 = i16 5000 ("x")
            n235 = Bundle("x"=w830, "x"=w830) -> (w831:cluster{"x":i16, "x":i16})  [unwired: 1 in]
            n236 = invoke class="Ctl" method="Move"(reference=w835, error in=w834, "position"=w831) -> (reference out=w832:refnum<vi>, error out=w833:errorcluster)  [unwired: 3 in, 4 out]
          }
          n237 = property class="ConPane"(reference=w615, error in=w605) -> (reference out=w604:refnum<vi>, error out=w613:errorcluster, "Ctrls[]"=w602:refnum<vi>[], "TermBnds[]"=w614:T5[])
          n238 = Bundle(w612, w612) -> (w610:cluster{i16, i16})  [unwired: 1 in]
          n239 = Bundle(w612, w611) -> (w609:cluster{i16, i16})  [unwired: 1 in]
          n240 = Bundle(w611, w611) -> (w608:cluster{i16, i16})  [unwired: 1 in]
          n241 = Bundle(w612, w611) -> (w607:cluster{i16, i16})  [unwired: 1 in]
          n242 = Build Array(w610, w609, w608, w607) -> (w606:cluster{i16, i16}[])
          n243 = Close Reference(reference=w604) -> ()  [unwired: 1 in, 1 out]
          n244 = for {
            tunnel: w614 -> [w799] mode=indexing
            tunnel: w602 -> [w775] mode=indexing
            tunnel: w606 -> [w789]
            shift-right: [w786] -> w603
            shift-left: w613 -> [w782]
            tunnel: [w781] -> w601 mode=indexing if=w777
            tunnel: [w780] -> w600 mode=indexing if=w776
            tunnel: [w767] -> w571 mode=indexing if=w765
            tunnel: [w766] -> w570 mode=indexing if=w764
            n245 = Unbundle By Name(w799) -> ("Left"=w796:i16, "Top"=w798:i16, "Right"=w797:i16, "Bottom"=w795:i16)
            n246 = Bundle("Left"=w796, "Top"=w798) -> (w791:cluster{"Left":i16, "Top":i16})  [unwired: 1 in]
            n247 = Bundle("Top"=w798, "Right"=w797) -> (w792:cluster{"Top":i16, "Right":i16})  [unwired: 1 in]
            n248 = Bundle("Right"=w797, "Bottom"=w795) -> (w793:cluster{"Right":i16, "Bottom":i16})  [unwired: 1 in]
            n249 = Bundle("Left"=w796, "Bottom"=w795) -> (w794:cluster{"Left":i16, "Bottom":i16})  [unwired: 1 in]
            n250 = Build Array(w791, w792, w793, w794) -> (w790:cluster{"Left":i16, "Bottom":i16}[])
            n251 = Equal?(x=w790, y=w789) -> (x = y?=w788:cluster{bool, bool}[])
            n252 = for {
              tunnel: w788 -> [w829] mode=indexing
              tunnel: [w827] -> w772 mode=indexing
              n253 = Cluster To Array(cluster=w829) -> (array=w828:bool[])
              n254 = And Array Elements(Boolean array=w828) -> (logical AND=w827:bool)
            }
            n255 = Not A Number/Path/Refnum?(number/path/refnum=w775) -> (NaN/Path/Refnum?=w773:bool)
            n256 = Select(t=bool[] [], s=w773, f=w772) -> (s? t:f=w774:bool[])
            n257 = Boolean Array To Number(Boolean array=w774) -> (number=w768:u32)
            n258 = Equal?(x=w768, y=u32 8) -> (x = y?=w777:bool)
            n259 = Equal?(x=w768, y=u32 4) -> (x = y?=w776:bool)
            n260 = Equal?(x=w768, y=u32 2) -> (x = y?=w765:bool)
            n261 = Equal?(x=w768, y=u32 1) -> (x = y?=w764:bool)
            n262 = Or Array Elements(Boolean array=w774) -> (logical OR=w787:bool)
            n263 = case shown="2" w768 {
              tunnel: [_ w804 w809 w814 w819] -> w785
              tunnel: [w800 w802 w807 w812 w817] -> w784
              tunnel: w775 -> [w800 w802 w807 w812 w817]
              tunnel: [w801 w803 w808 w813 w818] -> w783
              tunnel: w782 -> [w801 w803 w808 w813 w818]
              tunnel: [_ _ _ _ w817] -> w781
              tunnel: [_ _ _ w812 _] -> w780
              tunnel: [_ _ w807 _ _] -> w767
              tunnel: [_ w802 _ _ _] -> w766
              frame 0, Default {
              }
              frame 1 {
                n264 = Bundle("x"=i16 10, "x"=i16 20) -> (w804:cluster{"x":i16, "x":i16})  [unwired: 1 in]
              }
              frame 2 {
                n265 = Bundle("x"=i16 10000, "x"=i16 20) -> (w809:cluster{"x":i16, "x":i16})  [unwired: 1 in]
              }
              frame 4 {
                n266 = Bundle("x"=i16 10000, "x"=i16 10000) -> (w814:cluster{"x":i16, "x":i16})  [unwired: 1 in]
              }
              frame 8 {
                n267 = Bundle("x"=i16 10, "x"=i16 10000) -> (w819:cluster{"x":i16, "x":i16})  [unwired: 1 in]
              }
            }
            n268 = case shown="True" w787 {
              tunnel: w784 -> [_ w826]
              tunnel: w783 -> [w822 w825]
              tunnel: [w822 w824] -> w786
              tunnel: w785 -> [_ w823]
              frame False {
              }
              frame True {
                n269 = invoke class="Ctl" method="Move"(reference=w826, error in=w825, "position"=w823) -> (error out=w824:errorcluster)  [unwired: 3 in, 5 out]
              }
            }
          }
          n270 = Index Array(array=w601) -> (element=w540:refnum<vi>)  [unwired: 1 in]
          n271 = Index Array(array=w600) -> (element=w548:refnum<vi>)  [unwired: 1 in]
          n272 = Index Array(array=w571) -> (element=w564:refnum<vi>)  [unwired: 1 in]
          n273 = Index Array(array=w570) -> (element=w550:refnum<vi>)  [unwired: 1 in]
          n274 = for {
            tunnel: w616 -> [w870] mode=indexing
            tunnel: [w869] -> w546 mode=indexing if=w868
            tunnel: [w869] -> w543 mode=indexing if=w867
            shift-right: [w865] -> w552
            shift-left: w603 -> [w866]
            n275 = property class="Ctl"(reference=w870, error in=w866) -> (reference out=w869:refnum<vi>, error out=w865:errorcluster, "Indicator"=w867:bool)
            n276 = Not(x=w867) -> (.not. x?=w868:bool)
          }
          n277 = Not A Number/Path/Refnum?(number/path/refnum=w540) -> (NaN/Path/Refnum?=w551:bool)
          n278 = Not A Number/Path/Refnum?(number/path/refnum=w548) -> (NaN/Path/Refnum?=w549:bool)
          n279 = case shown="False" w551 {
            tunnel: w540 -> [w652 _]
            tunnel: [w651 _] -> w547
            frame False {
              n280 = property class="Ctl"(reference=w652) -> ("Label.Text"=w651:string)  [unwired: 1 in, 2 out]
            }
            frame True {
            }
          }
          n281 = case shown="False" w549 {
            tunnel: w548 -> [w650 _]
            tunnel: [w649 _] -> w544
            frame False {
              n282 = property class="Ctl"(reference=w650) -> ("Label.Text"=w649:string)  [unwired: 1 in, 2 out]
            }
            frame True {
            }
          }
          n283 = for {
            tunnel: w546 -> [w661] mode=indexing
            shift-right: [w654] -> w545
            shift-left: w552 -> [w660]
            tunnel: w547 -> [w658]
            shift-right: [w655] -> w538
            shift-left: w546 -> [w656]
            i -> [w653]
            n284 = property class="Ctl"(reference=w661, error in=w660) -> (error out=w654:errorcluster, "Label.Text"=w659:string)  [unwired: 1 out]
            n285 = Equal?(x=w659, y=w658) -> (x = y?=w657:bool)
            n286 = case shown="True" w657 {
              tunnel: w656 -> [w662 w667]
              tunnel: [w662 w664] -> w655
              tunnel: w653 -> [_ w666]
              frame False {
              }
              frame True {
                n287 = Delete From Array(array=w667, index=w666) -> (deleted portion=w663:refnum<vi>, array with subset deleted=w665:refnum<vi>[])  [unwired: 1 in]
                n288 = Build Array (concatenate)(w665, w663) -> (w664:refnum<vi>[])
              }
            }
          }
          n289 = Build Array(w540, w548) -> (w554:refnum<vi>[])
          n290 = for {
            tunnel: w543 -> [w642] mode=indexing
            shift-right: [w635] -> w542
            shift-left: w545 -> [w641]
            tunnel: w544 -> [w639]
            shift-right: [w636] -> w537
            shift-left: w543 -> [w637]
            i -> [w634]
            n291 = property class="Ctl"(reference=w642, error in=w641) -> (error out=w635:errorcluster, "Label.Text"=w640:string)  [unwired: 1 out]
            n292 = Equal?(x=w640, y=w639) -> (x = y?=w638:bool)
            n293 = case shown="True" w638 {
              tunnel: w637 -> [w643 w648]
              tunnel: [w643 w645] -> w636
              tunnel: w634 -> [_ w647]
              frame False {
              }
              frame True {
                n294 = Delete From Array(array=w648, index=w647) -> (deleted portion=w644:refnum<vi>, array with subset deleted=w646:refnum<vi>[])  [unwired: 1 in]
                n295 = Build Array (concatenate)(w646, w644) -> (w645:refnum<vi>[])
              }
            }
          }
          n296 = Build Array(w564, w550) -> (w556:refnum<vi>[])
          n297 = for {
            tunnel: w556 -> [w673] mode=indexing
            tunnel: [w673] -> w555 mode=indexing if=w671
            n298 = Not A Number/Path/Refnum?(number/path/refnum=w673) -> (NaN/Path/Refnum?=w672:bool)
            n299 = Not(x=w672) -> (.not. x?=w671:bool)
          }
          n300 = Array Size(array=w555) -> (size(s)=w568:i32)
          n301 = Equal?(x=2, y=w568) -> (x = y?=w567:bool)
          n302 = Equal To 0?(x=w568) -> (x = 0?=w566:bool)
          n303 = for {
            tunnel: w554 -> [w670] mode=indexing
            tunnel: [w670] -> w553 mode=indexing if=w668
            n304 = Not A Number/Path/Refnum?(number/path/refnum=w670) -> (NaN/Path/Refnum?=w669:bool)
            n305 = Not(x=w669) -> (.not. x?=w668:bool)
          }
          n306 = Or(x=w567, y=w566) -> (x .or. y?=w541:bool)
          n307 = case shown="False" w541 {
            tunnel: w542 -> [w705 w742]
            tunnel: w565 -> [w704 w741]
            tunnel: w564 -> [w706 _]
            tunnel: w550 -> [w707 _]
            tunnel: [w703 w742] -> w560
            tunnel: [w702 w741] -> w559
            tunnel: w537 -> [w701 _]
            tunnel: w538 -> [w700 _]
            frame False {
              n308 = Not A Number/Path/Refnum?(number/path/refnum=w707) -> (NaN/Path/Refnum?=w708:bool)
              n309 = case shown="False" w708 {
                tunnel: w707 -> [w724 _]
                tunnel: w706 -> [_ w727]
                tunnel: w705 -> [w723 w740]
                tunnel: w704 -> [w711 w728]
                tunnel: [w715 w732] -> w703
                tunnel: [w711 w728] -> w702
                tunnel: w701 -> [w709 _]
                tunnel: w700 -> [_ w725]
                frame False {
                  n310 = property class="Ctl"(reference=w724, error in=w723) -> (error out=w719:errorcluster, "MasterRect"=w722:T5)  [unwired: 1 out]
                  n311 = Unbundle By Name(w722) -> ("Bottom"=w721:i16)
                  n312 = Add(x=w721, y=i16 18) -> (x+y=w713:i16)
                  n313 = Index Array(array=w709) -> (element=w710:refnum<vi>)  [unwired: 1 in]
                  n314 = property class="Ctl"(reference=w710, error in=w719) -> (reference out=w717:refnum<vi>, error out=w716:errorcluster, "MasterRect"=w718:T5)
                  n315 = Unbundle By Name(w718) -> ("Left"=w714:i16)
                  n316 = Bundle("Left"=w714, w713) -> (w712:cluster{"Left":i16, i16})  [unwired: 1 in]
                  n317 = invoke class="Ctl" method="Move"(reference=w717, error in=w716, "position"=w712) -> (error out=w715:errorcluster)  [unwired: 3 in, 5 out]
                }
                frame True {
                  n318 = property class="Ctl"(reference=w727, error in=w740) -> (error out=w736:errorcluster, "MasterRect"=w739:T5)  [unwired: 1 out]
                  n319 = Unbundle By Name(w739) -> ("Bottom"=w738:i16)
                  n320 = Add(x=w738, y=i16 18) -> (x+y=w730:i16)
                  n321 = Index Array(array=w725) -> (element=w726:refnum<vi>)  [unwired: 1 in]
                  n322 = property class="Ctl"(reference=w726, error in=w736) -> (reference out=w734:refnum<vi>, error out=w733:errorcluster, "MasterRect"=w735:T5)
                  n323 = Unbundle By Name(w735) -> ("Left"=w731:i16)
                  n324 = Bundle("Left"=w731, w730) -> (w729:cluster{"Left":i16, i16})  [unwired: 1 in]
                  n325 = invoke class="Ctl" method="Move"(reference=w734, error in=w733, "position"=w729) -> (error out=w732:errorcluster)  [unwired: 3 in, 5 out]
                }
              }
            }
            frame True {
            }
          }
          n326 = Array Size(array=w555) -> (size(s)=w563:i32)
          n327 = Equal To 0?(x=w563) -> (x = 0?=w562:bool)
          n328 = case shown="True" w562 {
            tunnel: [w674 w678] -> w561
            tunnel: w560 -> [w674 w679]
            tunnel: w559 -> [w675 w676]
            tunnel: [w675 w676] -> w558
            tunnel: w538 -> [_ w683]
            tunnel: w537 -> [_ w682]
            frame False {
            }
            frame True {
              n329 = Index Array(array=w683) -> (element=w681:refnum<vi>)  [unwired: 1 in]
              n330 = Index Array(array=w682) -> (element=w680:refnum<vi>)  [unwired: 1 in]
              n331 = Build Array(w681, w680) -> (w677:refnum<vi>[])
              n332 = for {
                tunnel: w677 -> [w685] mode=indexing
                shift-right: [w687] -> w678
                shift-left: w679 -> [w688]
                i -> [w686]
                n333 = Not A Number/Path/Refnum?(number/path/refnum=w685) -> (NaN/Path/Refnum?=w684:bool)
                n334 = case shown="False" w684 {
                  tunnel: w688 -> [w698 w699]
                  tunnel: w685 -> [w697 _]
                  tunnel: w686 -> [w693 _]
                  tunnel: [w689 w699] -> w687
                  frame False {
                    n335 = Equal To 0?(x=w693) -> (x = 0?=w692:bool)
                    n336 = Select(t=i16 10 ("x"), s=w692, f=i16 5000 ("x")) -> (s? t:f=w694:i16)
                    n337 = Bundle("x"=w694, "x"=i16 20) -> (w695:cluster{"x":i16, "x":i16})  [unwired: 1 in]
                    n338 = invoke class="Ctl" method="Move"(reference=w697, error in=w698, "position"=w695) -> (error out=w689:errorcluster)  [unwired: 3 in, 5 out]
                  }
                  frame True {
                  }
                }
              }
            }
          }
          n339 = invoke class="Pnl" method="Make Selection"(reference=w558, error in=w561, "Objects"=w538) -> (reference out=w631:refnum<vi>, error out=w630:errorcluster)  [unwired: 1 in, 2 out]
          n340 = invoke class="Pnl" method="AlignSelection"(reference=w631, error in=w630, "Align Type"=T2."Left Edges") -> (reference out=w623:refnum<vi>, error out=w625:errorcluster)  [unwired: 1 in, 2 out]
          n341 = for {
            tunnel: w538 -> [w854] mode=indexing
            tunnel: [w857] -> w557 mode=indexing
            shift-right: [w855] -> w626
            shift-left: w625 -> [w856]
            n342 = Not A Number/Path/Refnum?(number/path/refnum=w854) -> (NaN/Path/Refnum?=w853:bool)
            n343 = case shown="False" w853 {
              tunnel: w854 -> [w862 _]
              tunnel: [w860 _] -> w857
              tunnel: w856 -> [w859 w863]
              tunnel: [w858 w863] -> w855
              frame False {
                n344 = property class="Ctl"(reference=w862, error in=w859) -> (error out=w858:errorcluster, "MasterRect"=w861:T5)  [unwired: 1 out]
                n345 = Unbundle By Name(w861) -> ("Right"=w860:i16)
              }
              frame True {
              }
            }
          }
          n346 = Array Max & Min(array=w557) -> (max value=w627:i16)  [unwired: 3 out]
          n347 = for {
            tunnel: w627 -> [w840]
            shift-right: [w838] -> w624
            shift-left: w626 -> [w839]
            tunnel: w537 -> [w836] mode=indexing
            n348 = Not A Number/Path/Refnum?(number/path/refnum=w836) -> (NaN/Path/Refnum?=w837:bool)
            n349 = case shown="False" w837 {
              tunnel: w840 -> [w851 _]
              tunnel: w836 -> [w849 _]
              tunnel: w839 -> [w848 w852]
              tunnel: [w843 w852] -> w838
              frame False {
                n350 = property class="Ctl"(reference=w849, error in=w848) -> (reference out=w841:refnum<vi>, error out=w842:errorcluster, "MasterRect"=w847:T5)
                n351 = Unbundle By Name(w847) -> ("Top"=w845:i16)
                n352 = Add(x=i16 20, y=w851) -> (x+y=w844:i16)
                n353 = Bundle(w844, "Top"=w845) -> (w846:cluster{i16, "Top":i16})  [unwired: 1 in]
                n354 = invoke class="Ctl" method="Move"(reference=w841, error in=w842, "position"=w846) -> (error out=w843:errorcluster)  [unwired: 3 in, 5 out]
              }
              frame True {
              }
            }
          }
          n355 = invoke class="Pnl" method="Make Selection"(reference=w623, error in=w624, "Objects"=w538) -> (reference out=w622:refnum<vi>, error out=w621:errorcluster)  [unwired: 1 in, 2 out]
          n356 = invoke class="Pnl" method="DistributeSelection"(reference=w622, error in=w621, "DistributeType"=w619) -> (reference out=w535:refnum<vi>, error out=w536:errorcluster)  [unwired: 1 in, 2 out]
          n357 = invoke class="Pnl" method="Make Selection"(reference=w535, error in=w536, "Objects"=w537) -> (reference out=w539:refnum<vi>, error out=w620:errorcluster)  [unwired: 1 in, 2 out]
          n358 = invoke class="Pnl" method="DistributeSelection"(reference=w539, error in=w620, "DistributeType"=w619) -> (reference out=w533:refnum<vi>, error out=w534:errorcluster)  [unwired: 1 in, 2 out]
          n359 = Array Size(array=w553) -> (size(s)=w599:i32)
          n360 = Equal?(x=2, y=w599) -> (x = y?=w597:bool)
          n361 = case shown="True" w597 {
            tunnel: w533 -> [w755 w763]
            tunnel: [w755 w762] -> w590
            tunnel: w534 -> [w754 w760]
            tunnel: [w754 w758] -> w589
            tunnel: w553 -> [_ w756]
            frame False {
            }
            frame True {
              n362 = invoke class="Pnl" method="Make Selection"(reference=w763, error in=w760, "Objects"=w756) -> (reference out=w761:refnum<vi>, error out=w759:errorcluster)  [unwired: 1 in, 2 out]
              n363 = invoke class="Pnl" method="AlignSelection"(reference=w761, error in=w759, "Align Type"=T2."Bottom Edges") -> (reference out=w762:refnum<vi>, error out=w758:errorcluster)  [unwired: 1 in, 2 out]
            }
          }
          n364 = for {
            tunnel: w538 -> [w753] mode=indexing
            shift-right: [w751] -> w587
            shift-left: w589 -> [w752]
            tunnel: [w749] -> w588 mode=indexing
            n365 = property class="Ctl"(reference=w753, error in=w752) -> (error out=w751:errorcluster, "MasterRect"=w750:T5)  [unwired: 1 out]
            n366 = Unbundle By Name(w750) -> ("Bottom"=w749:i16)
          }
          n367 = for {
            tunnel: w537 -> [w748] mode=indexing
            shift-right: [w746] -> w584
            shift-left: w587 -> [w747]
            tunnel: [w744] -> w586 mode=indexing
            tunnel: [w743] -> w585 mode=indexing
            n368 = property class="Ctl"(reference=w748, error in=w747) -> (error out=w746:errorcluster, "MasterRect"=w745:T5)  [unwired: 1 out]
            n369 = Unbundle By Name(w745) -> ("Right"=w744:i16, "Bottom"=w743:i16)
          }
          n370 = Array Max & Min(array=w586) -> (max value=w593:i16)  [unwired: 3 out]
          n371 = Build Array (concatenate)(w585, w588) -> (w596:i16[])
          n372 = Array Max & Min(array=w596) -> (max value=w592:i16)  [unwired: 3 out]
          n373 = Add(x=i16 10, y=w593) -> (x+y=w583:i16)
          n374 = Bundle("x"=w594, "x"=w594, w583, w592) -> (w591:cluster{"x":i16, "x":i16, i16, i16})  [unwired: 1 in]
          n375 = property class="VI"(reference=w595, error in=w584, "Front Panel.PanelBounds"=w591) -> (reference out=w581:refnum<vi>, error out=w579:errorcluster)
          n376 = invoke class="VI" method="FP.Center"(reference=w581, error in=w579) -> (reference out=w580:refnum<vi>, error out=w578:errorcluster)  [unwired: 1 in, 1 out]
          n377 = Build Array (concatenate)(w590, w538, w537, w602) -> (w628:refnum<vi>[])
          n378 = for {
            tunnel: w578 -> [_]
            tunnel: w628 -> [w864] mode=indexing
            n379 = Close Reference(reference=w864) -> ()  [unwired: 1 in, 1 out]
          }
          n380 = invoke class="VI" method="Save.Instrument"(reference=w580, error in=w578) -> (reference out=w572:refnum<vi>, error out=w577:errorcluster)  [unwired: 4 in, 4 out]
          n381 = Close Reference(reference=w572) -> ()  [unwired: 1 in, 1 out]
        }
      }
    }
    frame Error {
    }
  }
  "error out" <- w5
  "CS++Actor out" <- w3
